vi "subBTInitRoutine.vi"(7 "Reorder Array":i32[](array[numeric]), 8 "error in (no error)":errorcluster, 10 "Number of retries":i32, 11 "No. of Wiimotes":i32) -> (0 "error out":errorcluster, 3 "Number of wiimotes paired":i32)   [LabVIEW 2009]
uses:
  Action Engines/AE Access VIs/AE - Bluetooth Connect All.vi
  Action Engines/AE Access VIs/AE - Bluetooth Initialise.vi
  Action Engines/AE Access VIs/AE - Bluetooth Pair All.vi
  Action Engines/AE Access VIs/AE - Bluetooth Reorder.vi
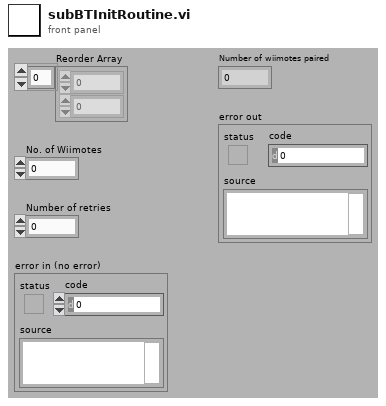
[diagram p1: front panel]
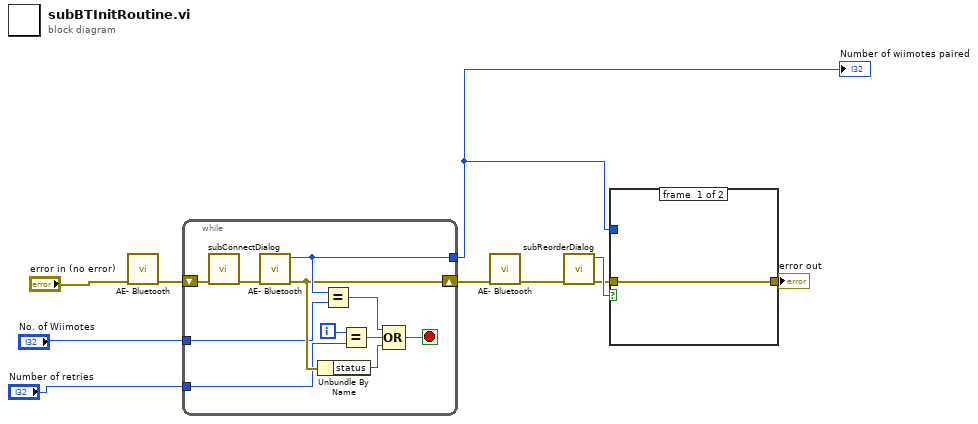
[diagram p0: block diagram]
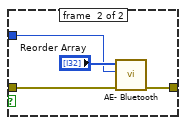
[diagram p2: hidden frame]
diagram:
  n1 = call-poly "AE- Bluetooth.vi"("error in (no error)"="error in (no error)") -> ("error out"=w2:errorcluster)  [unwired: 10 in]
  n2 = while {
    tunnel: [w15] -> w8
    shift-right: [w14] -> w3
    shift-left: w2 -> [w17]
    tunnel: "No. of Wiimotes" -> [w12]
    tunnel: "Number of retries" -> [w11]
    i -> [w20]
    stop <- w18 stop-if-true
    n3 = call "subConnectDialog.vi"("error in (no error)"=w17) -> ("error out"=w16:errorcluster)  [unwired: 10 in]
    n4 = call-poly "AE- Bluetooth.vi"("error in (no error)"=w16) -> ("error out"=w14:errorcluster, "Number of wiimotes paired"=w15:i32)  [unwired: 9 in]
    n5 = Unbundle By Name(w14) -> ("status"=w13:bool)
    n6 = Equal?(x=w15, y=w12) -> (x = y?=w21:bool)
    n7 = Equal?(x=w20, y=w11) -> (x = y?=w19:bool)
    n8 = Compound Arithmetic op=OR(w21, w19, w13) -> (w18:bool)
  }
  "Number of wiimotes paired" <- w8
  n9 = call-poly "AE- Bluetooth.vi"("error in (no error)"=w3) -> ("error out"=w6:errorcluster)  [unwired: 9 in, 1 out]
  n10 = call "subReorderDialog.vi"("error in"=w6) -> ("error out"=w5:errorcluster, "T button?"=w7:bool)  [unwired: 9 in]
  n11 = case shown="True" w7 {
    tunnel: w5 -> [w22 w25]
    tunnel: [w22 w26] -> w4
    tunnel: w8 -> [_ w23]
    frame #0 {
    }
    frame #1 {
      n12 = call-poly "AE- Bluetooth.vi"("error in (no error)"=w25, "No. of Wiimotes Paired"=w23, "Reorder Array"="Reorder Array") -> ("error out"=w26:errorcluster)  [unwired: 8 in]
    }
  }
  "error out" <- w4
